vi "run sipper pump.vi"(2 "pump time":dbl[unit] format="%.2f", 3 "GPIB in":string="18") -> (1 "GPIB out":string="18")   [LabVIEW 2015]
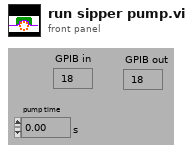
[diagram p1: front panel]
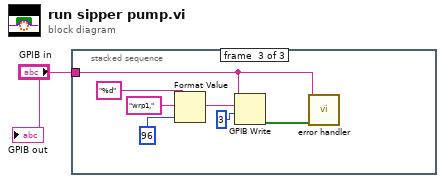
[diagram p0: block diagram]
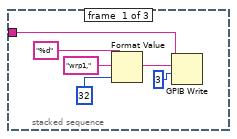
[diagram p2: hidden frame]
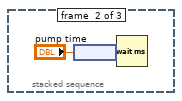
[diagram p3: hidden frame]
diagram:
  n1 = stacked-sequence {
    tunnel: "GPIB in" -> [w3 _ w11]
    frame #0 {
      n2 = Format Value(string ("")="wrp1,", format string="%d", value (0)=32) -> (output string=w4:string)
      n3 = GPIB Write(0:w3, 1:w4, 2:3) -> ()  [unwired: 2 in, 2 out]
    }
    frame #1 {
      n4 = node("pump time") -> (w8:dbl)
      n5 = Wait (ms)(milliseconds to wait=w8) -> ()  [unwired: 1 out]
    }
    frame #2 {
      n6 = Format Value(string ("")="wrp1,", format string="%d", value (0)=96) -> (output string=w13:string)
      n7 = GPIB Write(0:w11, 1:w13, 2:3) -> (5:w10:bool[])  [unwired: 2 in, 1 out]
      n8 = call "error handler.vi"("status array"=w10, "GPIB in"=w11) -> ()  [unwired: 3 in, 3 out]
    }
  }
  "GPIB out" <- "GPIB in"
